vi "PCE_ANSWER-error-handler(numU32).vi"(1 "Boolean array":u32, 2 "Serial?":bool) -> (0 "PCE answer":string)   [LabVIEW 2010]
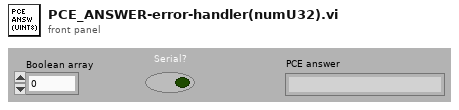
[diagram p1: front panel]
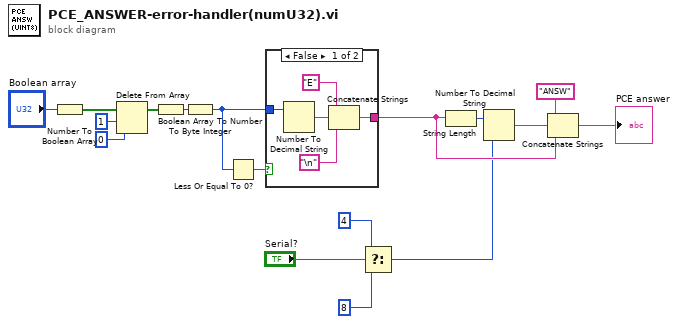
[diagram p0: block diagram]
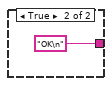
[diagram p2: hidden frame]
diagram:
  n1 = Number To Boolean Array(number="Boolean array") -> (Boolean array=w5:bool[])
  n2 = Delete From Array(array=w5, length=1, index=0) -> (array with subset deleted=w6:bool[])  [unwired: 1 out]
  n3 = Boolean Array To Number(Boolean array=w6) -> (number=w15:u32)
  n4 = To Byte Integer(number=w15) -> (8bit integer=w7:i8)
  n5 = Less Or Equal To 0?(x=w7) -> (x <= 0?=w8:bool)
  n6 = case shown="False" w8 {
    tunnel: w7 -> [w20 _]
    tunnel: [w19 "OK\n"] -> w11
    frame False {
      n7 = Number To Decimal String(number=w20) -> (decimal integer string=w22:string)  [unwired: 1 in]
      n8 = Concatenate Strings("E" ("string"), w22, "\n" ("string")) -> (w19:string)
    }
    frame True {
    }
  }
  n9 = Select(t=i16 4 ("width (-)"), s="Serial?", f=i16 8 ("width (-)")) -> (s? t:f=w3:i16)
  n10 = String Length(string=w11) -> (length=w12:i32)
  n11 = Number To Decimal String(number=w12, width (-)=w3) -> (decimal integer string=w10:string)
  n12 = Concatenate Strings("ANSW" ("string"), w10, w11) -> (→"PCE answer":string)
